vi "Safe Image Get Image.vi"(6 "Video Mode":i32, 7 "Wait":bool, 8 "error in":errorcluster, 9 "Operation":T3(ring), 10 "Image In":T1, 11 "Session In":T2) -> (0 "error out":errorcluster, 1 "Image Data String":string, 2 "Image Out":T1, 3 "Session Out":T2)   [LabVIEW 2017]
doc: "For USB cameras, we use a subVI to prevent mode changes while retrieving images. This subVI also redoes the connection on some errors, trying to deal with a disconnect/reconnect of a USB camera."
uses:
  <vilib>/userdefined/High Color/IMAQdx.ctl
  <vilib>/vision/Image Controls.llb/IMAQ Image.ctl
  <vilib>/vision/driver/IMAQdx.llb/IMAQdx Buffer Number Mode.ctl
  <resource>/objmgr/imaqdx.rc
  <vilib>/vision/driver/NI_Vision_Acquisition_Software.lvlib
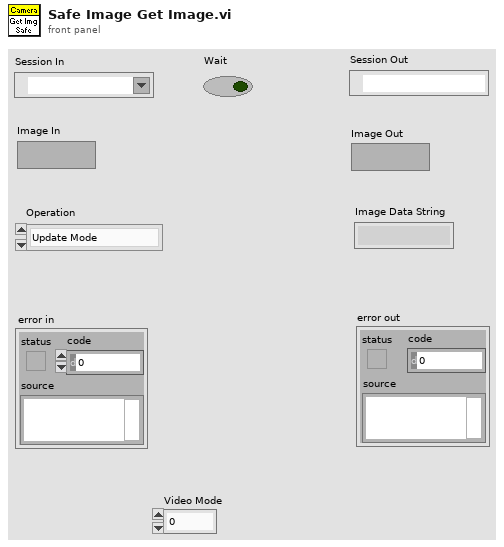
[diagram p1: front panel]
types:
  T1 = typedef "IMAQ Image.ctl" = refnum<image>
  T2 = typedef "IMAQdx.ctl" = refnum<k21>
  T3 = enum16{"Update Mode", "Get Image", "Get Image Data"}
  T4 = typedef "NI_Vision_Acquisition_Software.lvlib/IMAQdx Buffer Number Mode.ctl" = enum32{"Next", "Last", "Buffer Number", "Every", "Last New"}
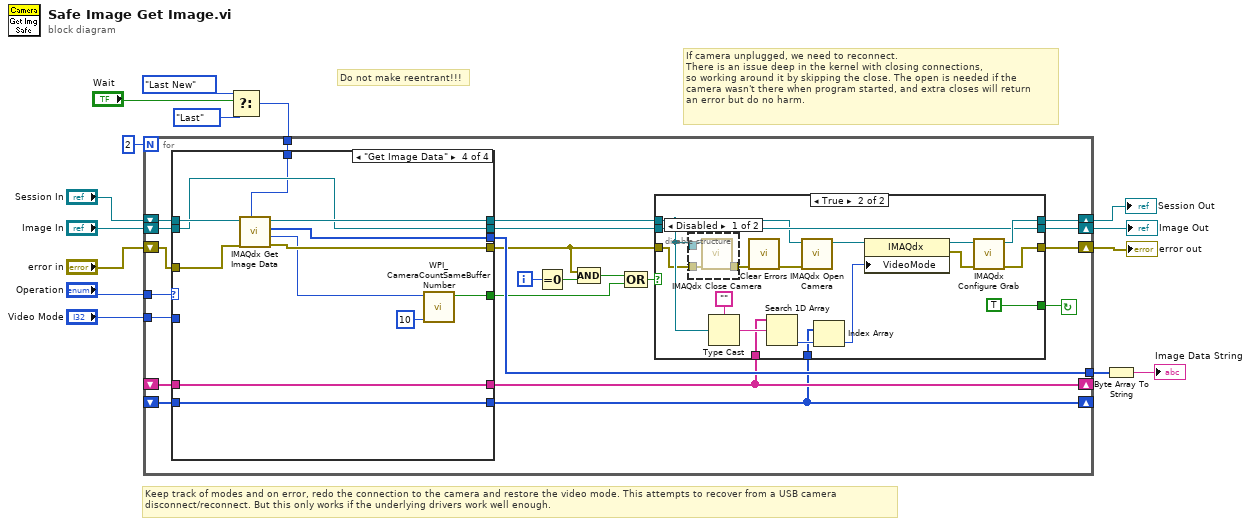
[diagram p0: block diagram]
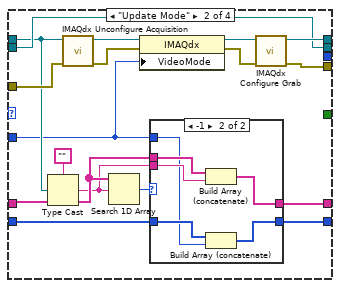
[diagram p5: hidden frame]
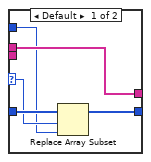
[diagram p6: hidden frame]
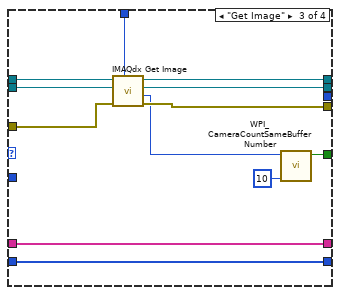
[diagram p7: hidden frame]
diagram:
  # "Do not make reentrant!!!"
  # "If camera unplugged, we need to reconnect.\nThere is an issue deep in the kernel with closing connections,\nso working around it by skipping the close. The open is needed if the\ncamera wasn't there when program started, and extra closes will return\nan error but do no harm."
  # "Keep track of modes and on error, redo the connection to the camera and restore the video mode. This attempts to recover from a USB camera\ndisconnect/reconnect. But this only works if the underlying drivers work well enough."
  n1 = Select(t=IMAQdx_Buffer_Number_Mode."Last New" ("Buffer Number Mode (Next)"), s="Wait", f=IMAQdx_Buffer_Number_Mode."Last" ("Buffer Number Mode (Next)")) -> (s? t:f=w1:T4)
  n2 = for {
    N: 2 -> [_]
    tunnel: "Operation" -> [w38]
    tunnel: "Video Mode" -> [w37]
    tunnel: [w33] -> w11
    shift-right: [w28] -> w9
    shift-left: "Session In" -> [w36]
    shift-right: [w30] -> w6
    shift-left: "Image In" -> [w35]
    shift-right: [w32] -> w5
    shift-left: "error in" -> [w34]
    shift-right: [w24] -> _
    shift-left: _ -> [w26]
    shift-right: [w23] -> _
    shift-left: _ -> [w25]
    tunnel: w1 -> [w19]
    i -> [w22]
    stop <- w27 continue-if-true
    n3 = case shown="\"Get Image Data\"" w38 {
      tunnel: w36 -> [w66 w72 w102 w115]
      tunnel: [w66 w81 w99 w117] -> w29
      tunnel: [w65 w79 w101 w116] -> w21
      tunnel: w37 -> [_ w68 _ _]
      tunnel: w35 -> [w64 w76 w103 w113]
      tunnel: [w64 w76 w100 w113] -> w31
      tunnel: [_ _ _ w118] -> w33
      tunnel: w34 -> [w65 w77 w104 w114]
      tunnel: w26 -> [w63 w74 w106 w112]
      tunnel: w25 -> [w62 w73 w105 w111]
      tunnel: [w63 w69 w106 w112] -> w24
      tunnel: [w62 w67 w105 w111] -> w23
      tunnel: w19 -> [_ _ w98 w110]
      tunnel: [_ _ w96 w107] -> w16
      frame Default {
      }
      frame "Update Mode" {
        n4 = Type Cast(type="", x=w72) -> (*(type *) &x=w70:string)
        n5 = call <vilib>:"IMAQdx Unconfigure Acquisition.vi"("error in"=w77, "Session In"=w72) -> ("error out"=w78:errorcluster, "Session Out"=w83:T2)  [unwired: 8 in]
        n6 = Search 1D Array(1D array=w74, element=w70) -> (index of element=w75:i32)  [unwired: 1 in]
        n7 = property class="IMAQdx"(reference=w83, error in=w78, "VideoMode"=w68) -> (reference out=w82:T2, error out=w80:errorcluster)
        n8 = case shown="-1" w75 {
          selector: w75 -> [w86 _]
          tunnel: w74 -> [w88 w94]
          tunnel: w73 -> [w87 w91]
          tunnel: w70 -> [_ w93]
          tunnel: [w88 w92] -> w69
          tunnel: w68 -> [w85 w89]
          tunnel: [w84 w90] -> w67
          frame Default {
            n9 = Replace Array Subset(array=w87, new element=w85, index=w86) -> (w84:i32[])
          }
          frame -1 {
            n10 = Build Array (concatenate)(w94, w93) -> (w92:string[])
            n11 = Build Array (concatenate)(w91, w89) -> (w90:i32[])
          }
        }
        n12 = call <vilib>:"IMAQdx Configure Grab.vi"("error in"=w80, "Session In"=w82) -> ("error out"=w79:errorcluster, "Session Out"=w81:T2)  [unwired: 8 in]
      }
      frame "Get Image" {
        n13 = call <vilib>:"IMAQdx Get Image.vi"("Buffer Number Mode (Next)"=w98, "error in"=w104, "Image In"=w103, "Session In"=w102) -> ("error out"=w101:errorcluster, "Buffer Number Out"=w97:u32, "Image Out"=w100:T1, "Session Out"=w99:T2)  [unwired: 4 in]
        n14 = call <vilib>:"WPI_CameraCountSameBufferNumber.vi"("Duplicates"=u32 10, "Number"=w97) -> ("Same"=w96:bool)  [unwired: 9 in]
      }
      frame "Get Image Data" {
        n15 = call <vilib>:"IMAQdx Get Image Data.vi"("Buffer Number Mode (Next)"=w110, "error in"=w114, "Session In"=w115) -> ("error out"=w116:errorcluster, "Buffer Number Out"=w109:u32, "Image Data Array"=w118:u8[], "Session Out"=w117:T2)  [unwired: 5 in]
        n16 = call <vilib>:"WPI_CameraCountSameBufferNumber.vi"("Duplicates"=u32 10, "Number"=w109) -> ("Same"=w107:bool)  [unwired: 9 in]
      }
    }
    n17 = Equal To 0?(x=w22) -> (x = 0?=w20:bool)
    n18 = Compound Arithmetic op=AND(w21, w20) -> (w18:bool)
    n19 = Compound Arithmetic op=OR(w18, w16) -> (w17:bool)
    n20 = case shown="True" w17 {
      tunnel: [w39 w42] -> w32
      tunnel: w31 -> [w41 w55]
      tunnel: [w41 w55] -> w30
      tunnel: w29 -> [w40 w49]
      tunnel: [w40 w56] -> w28
      tunnel: [_ TRUE] -> w27
      tunnel: w24 -> [_ w47]
      tunnel: w23 -> [_ w45]
      tunnel: w21 -> [w39 w43]
      frame False {
      }
      frame True {
        n21 = disable-structure shown="Disabled" {
          disable-tunnel: [w61 _] -> w58
          disable-tunnel: w49 -> [w60 _]
          disable-tunnel: w43 -> [w59 _]
          frame Disabled {
            n22 = call <vilib>:"IMAQdx Close Camera.vi"("error in"=w59, "Session In"=w60) -> ("error out"=w61:errorcluster)  [unwired: 9 in]
          }
          frame Enabled {
          }
        }
        n23 = Type Cast(type="", x=w49) -> (*(type *) &x=w48:string)
        n24 = call <vilib>:"Clear Errors.vi"("error in (no error)"=w58) -> ("error out"=w57:errorcluster)  [unwired: 5 in, 1 out]
        n25 = Search 1D Array(1D array=w47, element=w48) -> (index of element=w46:i32)  [unwired: 1 in]
        n26 = call <vilib>:"IMAQdx Open Camera.vi"("error in"=w57, "Session In"=w49) -> ("Session Out"=w53:T2)  [unwired: 8 in, 1 out]
        n27 = Index Array(array=w45, index=w46) -> (element=w44:i32)
        n28 = property class="IMAQdx"(reference=w53, "VideoMode"=w44) -> (reference out=w52:T2, error out=w51:errorcluster)  [unwired: 1 in]
        n29 = call <vilib>:"IMAQdx Configure Grab.vi"("error in"=w51, "Session In"=w52) -> ("error out"=w42:errorcluster, "Session Out"=w56:T2)  [unwired: 8 in]
      }
    }
  }
  "Session Out" <- w9
  "Image Out" <- w6
  "error out" <- w5
  n30 = Byte Array To String(unsigned byte array=w11) -> (string=→"Image Data String":string)
